vi "Tear Down Clock Discipline.vi"(8 "error in (no error)":errorcluster, 11 "RT Data Cluster in":T1={"Timekeeper hdl"="", "clkDisc session"=variant, "Compiled Data"={"SyncMod?"=FALSE, "SyncMod"="", "ConnectionSettings"={"Mode"=enum."Generate sample clock", "pxitrig"=FALSE, "pfi0"=FALSE, "pfi1"=FALSE, "pfi2"=FALSE, "External Pin"=enum."PFI0", "Routes"=[]}, "TimeKeeper"="", "ScanOffset(%)"=0.0, "StartDelay(s)"=0, "Time Ref Settings"={"Time Reference"=enum."GPS", "Priority 1"=0, "Priority 2"=0, "IRIG type"=enum."IRIGB AM", "Terminal"="", "PPSSetTime"=FALSE, "Start Time"=timestamp(0 s since 1904-01-01)}, "FIFO Locations"={"BoardTime"=[], "Status"=[]}}, "OutputsData"=[], "OutputsFIFO"=refnum, "Scan Period"=0, "Timekeeper type"=enum."6683", "SyncMod type"=enum."6683", "SyncMod hdl"=""} {"Compiled Data"."Time Ref Settings"."Priority 2" min=0 max=255; "Compiled Data"."Time Ref Settings"."Priority 1" min=0 max=255}) -> (0 "error out":errorcluster, 3 "RT Data Cluster out":T1={"Timekeeper hdl"="", "clkDisc session"=variant, "Compiled Data"={"SyncMod?"=FALSE, "SyncMod"="", "ConnectionSettings"={"Mode"=enum."Generate sample clock", "pxitrig"=FALSE, "pfi0"=FALSE, "pfi1"=FALSE, "pfi2"=FALSE, "External Pin"=enum."PFI0", "Routes"=[]}, "TimeKeeper"="", "ScanOffset(%)"=0.0, "StartDelay(s)"=0, "Time Ref Settings"={"Time Reference"=enum."GPS", "Priority 1"=0, "Priority 2"=0, "IRIG type"=enum."IRIGB AM", "Terminal"="", "PPSSetTime"=FALSE, "Start Time"=timestamp(0 s since 1904-01-01)}, "FIFO Locations"={"BoardTime"=[], "Status"=[]}}, "OutputsData"=[], "OutputsFIFO"=refnum, "Scan Period"=0, "Timekeeper type"=enum."6683", "SyncMod type"=enum."6683", "SyncMod hdl"=""} {"Compiled Data"."Time Ref Settings"."Priority 2" min=0 max=255; "Compiled Data"."Time Ref Settings"."Priority 1" min=0 max=255})   [LabVIEW 2015, in "Chassis TimeSync Engine.lvlib"]
uses:
  Chassis TimeSync Engine.lvlib
  RT Data Cluster.ctl
  mdevClkDisc.llb/_clkDisc_session.ctl
  Shared/Compiled Data.ctl
  Shared/Connection Settings.ctl
  Shared/Mode.ctl
  Shared/External Pin.ctl
  Shared/Routes.ctl
  Shared/Route.ctl
  Shared/Time Ref Settings.ctl
  Shared/Time Reference.ctl
  Shared/IRIG Type.ctl
  timekeeper type.ctl
  Timekeeper Route Pin.ctl
  Shared/Chassis TimeSync Shared.lvlib
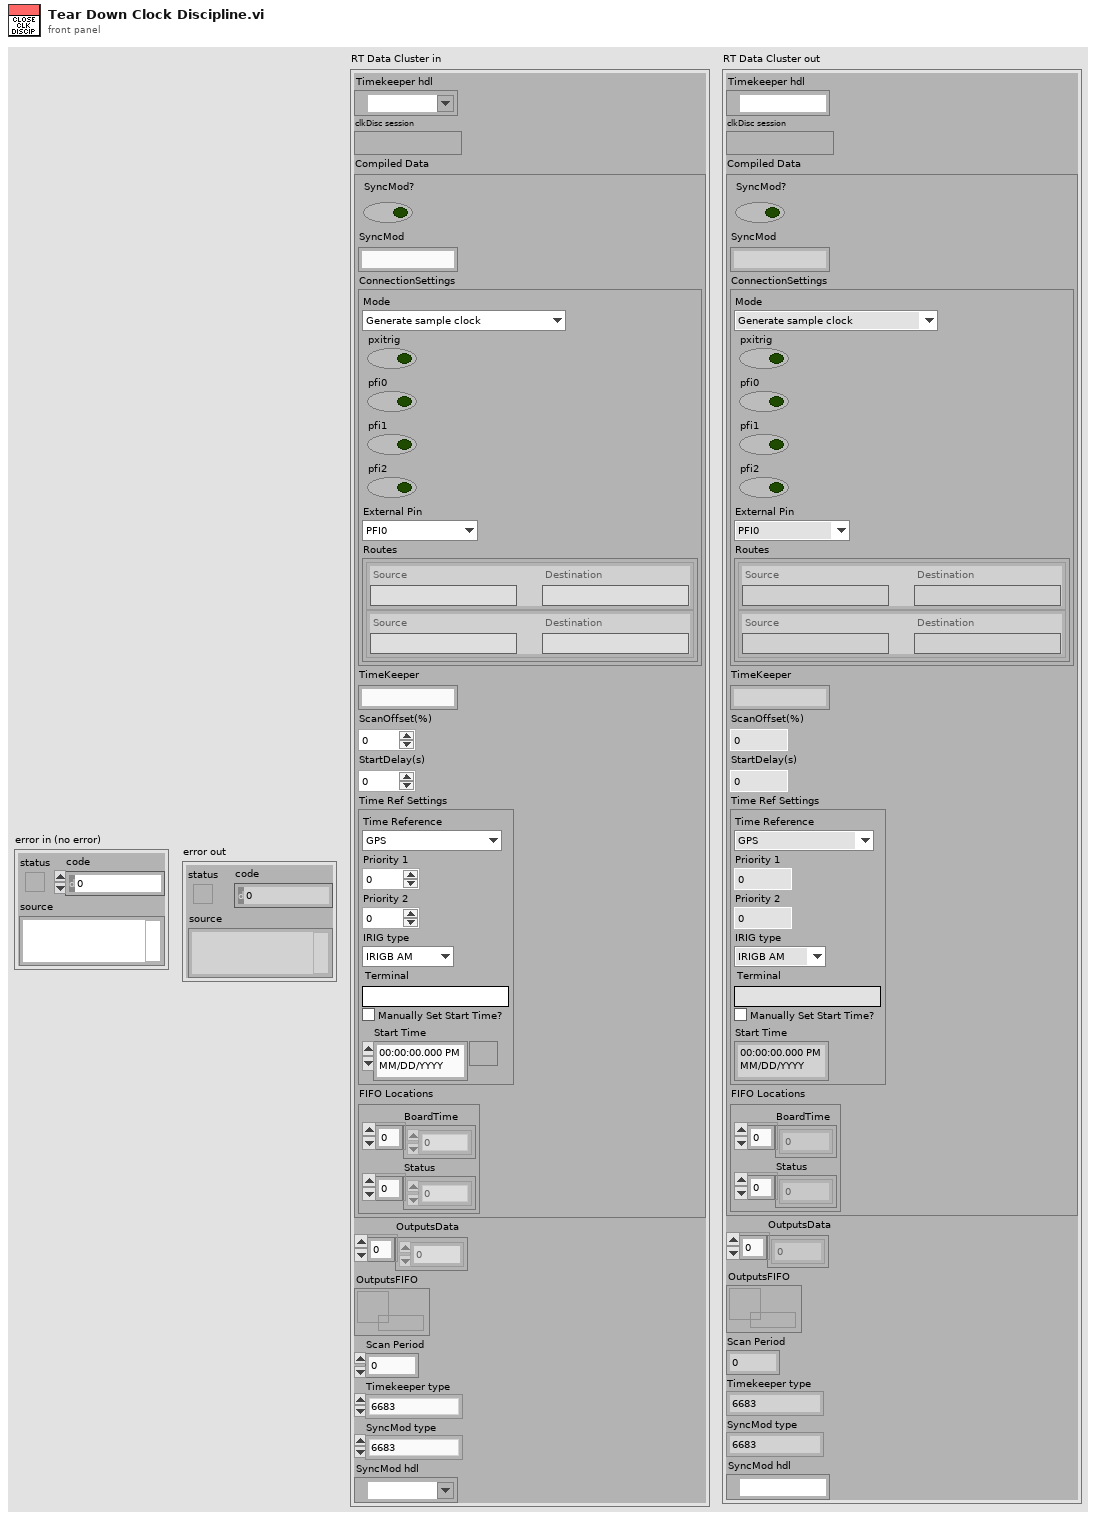
[diagram p1: front panel]
types:
  T1 = typedef "Chassis TimeSync Engine.lvlib/RT Data Cluster.ctl" = cluster{"Timekeeper hdl":refnum<k15>, "clkDisc session":T2, "Compiled Data":T3, "OutputsData":dbl[], "OutputsFIFO":refnum<k33>, "Scan Period":u32, "Timekeeper type":T12, "SyncMod type":T12, "SyncMod hdl":refnum<k15>}
  T2 = typedef "_clkDisc_session.ctl" = variant
  T3 = typedef "Chassis TimeSync Shared.lvlib/Compiled Data.ctl" = cluster{"SyncMod?":bool, "SyncMod":string, "ConnectionSettings":T4, "TimeKeeper":string, "ScanOffset(%)":dbl, "StartDelay(s)":u16, "Time Ref Settings":T9, "FIFO Locations":cluster{"BoardTime":i32[], "Status":i32[]}}
  T4 = typedef "Chassis TimeSync Shared.lvlib/Connection Settings.ctl" = cluster{"Mode":T5, "pxitrig":bool, "pfi0":bool, "pfi1":bool, "pfi2":bool, "External Pin":T6, "Routes":T7}
  T5 = typedef "Chassis TimeSync Shared.lvlib/Mode.ctl" = enum16{"Generate sample clock", "Route sample clock out of chassis", "Route sample clock into chassis", "Custom routes"}
  T6 = typedef "Chassis TimeSync Shared.lvlib/External Pin.ctl" = enum16{"PFI0", "PFI1", "PFI2"}
  T7 = typedef "Chassis TimeSync Shared.lvlib/Routes.ctl" = T8[]
  T8 = typedef "Chassis TimeSync Shared.lvlib/Route.ctl" = cluster{"Source":string, "Destination":string}
  T9 = typedef "Chassis TimeSync Shared.lvlib/Time Ref Settings.ctl" = cluster{"Time Reference":T10, "Priority 1":i32, "Priority 2":i32, "IRIG type":T11, "Terminal":string, "PPSSetTime":bool, "Start Time":timestamp}
  T10 = typedef "Chassis TimeSync Shared.lvlib/Time Reference.ctl" = enum16{"GPS", "IRIG", "PPS", "1588 Ordinary Clock", "PXI Chassis Clock", "Free Running (Internal)"}
  T11 = typedef "Chassis TimeSync Shared.lvlib/IRIG Type.ctl" = enum16{"IRIGB DC", "IRIGB AM"}
  T12 = typedef "Chassis TimeSync Engine.lvlib/timekeeper type.ctl" = enum16{"6683", "6683H", "6682", "6682H", "non-timekeeper", "timekeeper"}
  T13 = typedef "Chassis TimeSync Engine.lvlib/Timekeeper Route Pin.ctl" = enum16{"TTL0", "PFI0", "PFI1", "PFI2", "PXI_Clk10", "PXI_Clk10_In", "BoardClk", "ClkOut", "Oscillator"}
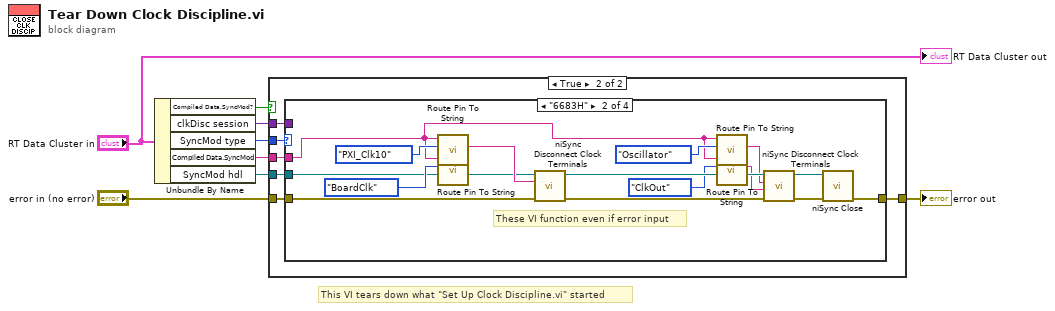
[diagram p0: block diagram]
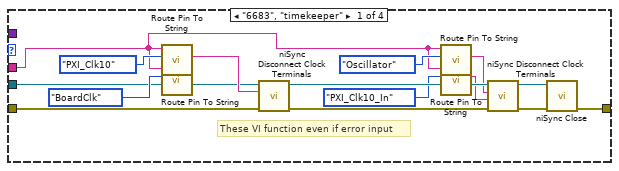
[diagram p3: hidden frame]
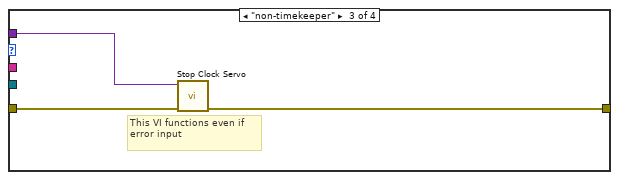
[diagram p4: hidden frame]
diagram:
  # "This VI tears down what \"Set Up Clock Discipline.vi\" started"
  n1 = Unbundle By Name("RT Data Cluster in") -> ("Compiled Data.SyncMod?"=w8:bool, "clkDisc session"=w6:T2, "SyncMod type"=w3:T12, "Compiled Data.SyncMod"=w1:string, "SyncMod hdl"=w2:refnum<k15>)
  n2 = case shown="True" w8 {
    tunnel: "error in (no error)" -> [w9 w15]
    tunnel: [w9 w14] -> w4
    tunnel: w6 -> [_ w13]
    tunnel: w3 -> [_ w12]
    tunnel: w2 -> [_ w10]
    tunnel: w1 -> [_ w11]
    frame False {
    }
    frame True {
      n3 = case shown="\"6683H\"" w12 {
        tunnel: w15 -> [w28 w43 w48 w49]
        tunnel: [w27 w42 w47 w49] -> w14
        tunnel: w13 -> [_ _ w46 _]
        tunnel: w11 -> [w18 w33 _ _]
        tunnel: w10 -> [w25 w40 _ _]
        frame "6683", "timekeeper" {
          # "These VI function even if error input"
          n4 = call "Route Pin To String.vi"("Pin"=Timekeeper_Route_Pin."PXI_Clk10", "Module"=w18) -> ("String"=w26:string)  [unwired: 9 in]
          n5 = call "Route Pin To String.vi"("Pin"=Timekeeper_Route_Pin."BoardClk", "Module"=w18) -> ()  [unwired: 9 in, 1 out]
          n6 = call <instrlib>:"niSync Disconnect Clock Terminals.vi"("error in (no error)"=w28, "source terminal"=w26, "instrument handle"=w25) -> ("error out"=w23:errorcluster, "instrument handle out"=w24:refnum<k15>)  [unwired: 7 in]
          n7 = call "Route Pin To String.vi"("Pin"=Timekeeper_Route_Pin."Oscillator", "Module"=w18) -> ("String"=w17:string)  [unwired: 9 in]
          n8 = call "Route Pin To String.vi"("Pin"=Timekeeper_Route_Pin."PXI_Clk10_In", "Module"=w18) -> ("String"=w16:string)  [unwired: 9 in]
          n9 = call <instrlib>:"niSync Disconnect Clock Terminals.vi"("error in (no error)"=w23, "destination terminal"=w16, "source terminal"=w17, "instrument handle"=w24) -> ("error out"=w22:errorcluster, "instrument handle out"=w21:refnum<k15>)  [unwired: 6 in]
          n10 = call <instrlib>:"niSync Close.vi"("error in (no error)"=w22, "instrument handle"=w21) -> ("error out"=w27:errorcluster)  [unwired: 9 in]
        }
        frame "6683H" {
          # "These VI function even if error input"
          n11 = call "Route Pin To String.vi"("Pin"=Timekeeper_Route_Pin."PXI_Clk10", "Module"=w33) -> ("String"=w41:string)  [unwired: 9 in]
          n12 = call "Route Pin To String.vi"("Pin"=Timekeeper_Route_Pin."BoardClk", "Module"=w33) -> ()  [unwired: 9 in, 1 out]
          n13 = call <instrlib>:"niSync Disconnect Clock Terminals.vi"("error in (no error)"=w43, "source terminal"=w41, "instrument handle"=w40) -> ("error out"=w38:errorcluster, "instrument handle out"=w39:refnum<k15>)  [unwired: 7 in]
          n14 = call "Route Pin To String.vi"("Pin"=Timekeeper_Route_Pin."Oscillator", "Module"=w33) -> ("String"=w32:string)  [unwired: 9 in]
          n15 = call "Route Pin To String.vi"("Pin"=Timekeeper_Route_Pin."ClkOut", "Module"=w33) -> ("String"=w31:string)  [unwired: 9 in]
          n16 = call <instrlib>:"niSync Disconnect Clock Terminals.vi"("error in (no error)"=w38, "destination terminal"=w31, "source terminal"=w32, "instrument handle"=w39) -> ("error out"=w37:errorcluster, "instrument handle out"=w36:refnum<k15>)  [unwired: 6 in]
          n17 = call <instrlib>:"niSync Close.vi"("error in (no error)"=w37, "instrument handle"=w36) -> ("error out"=w42:errorcluster)  [unwired: 9 in]
        }
        frame "non-timekeeper" {
          # "This VI functions even if error input"
          n18 = call "Stop Clock Servo.vi"("error (in)"=w48, "clkDisc session (in)"=w46) -> ("error (out)"=w47:errorcluster)  [unwired: 5 in]
        }
        frame "6682", "6682H" {
          # "This would have thrown an error in Set Up Clock Discipline. Pass through error"
        }
      }
    }
  }
  "error out" <- w4
  "RT Data Cluster out" <- "RT Data Cluster in"
